vi "Handle.vi"(7 "Actor in":refnum<class "Actor.lvclass">, 11 "Teardown State in":refnum<class "Teardown State.lvclass">) -> (2 "Destroy?":bool, 5 "Actor out":refnum<class "Actor.lvclass">)   [LabVIEW 2021, in "jettl.lvlib" / "jettl Queue Actor.lvlib" / "Teardown State.lvclass"]
uses:
  Teardown State.lvclass
  Actor/Actor/Actor.lvclass
  Actor/Msgs/Teardown/Teardown Msg/Teardown Msg.lvclass
  C:/git/jettl/src/Actor/Msg/Msg.lvclass
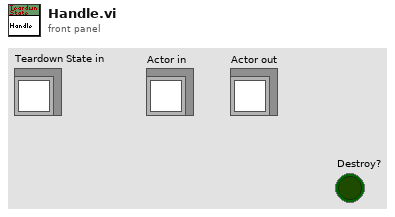
[diagram p1: front panel]
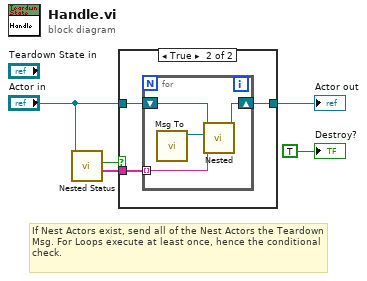
[diagram p0: block diagram]
diagram:
  # "If Nest Actors exist, send all of the Nest Actors the Teardown Msg. For Loops execute at least once, hence the conditional check."
  n1 = call-dynamic "Nested Status.vi"("Actor in"="Actor in") -> ("Nested Aliases"=w1:string[], "Any Exist?"=w2:bool)  [unwired: 8 in, 1 out]
  n2 = case shown="True" w2 {
    tunnel: [w6 w9] -> w4
    tunnel: "Actor in" -> [w6 w8]
    tunnel: w1 -> [_ w7]
    frame False {
    }
    frame True {
      n3 = for {
        tunnel: w7 -> [w12] mode=indexing
        shift-right: [w10] -> w9
        shift-left: w8 -> [w11]
        n4 = call "Msg To.vi"() -> ("Teardown Msg out"=w13:refnum<class "Teardown Msg.lvclass">)  [unwired: 11 in]
        n5 = call-dynamic "Nested.vi"("Alias"=w12, "Msg"=w13, "Actor in"=w11) -> ("Actor out"=w10:refnum<class "Actor.lvclass">)  [unwired: 8 in]
      }
    }
  }
  "Actor out" <- w4
  "Destroy?" <- TRUE ("Destroy?")
